vi "WaitForReceipt.vi"(8 "error in (no error)":errorcluster, 9 "timeout in ms (10000)":i32=10000, 11 "STOMP in":refnum<class "STOMP.lvclass">) -> (0 "error out":errorcluster, 2 "receipt":T1, 3 "STOMP out":refnum<class "STOMP.lvclass">)   [LabVIEW 2017, in "LabVIEW STOMP.lvlib" / "STOMP.lvclass"]
uses:
  STOMP.lvclass
  Typedefs/Type_ServerFrame.ctl
  Typedefs/Type_ServerFrameType.ctl
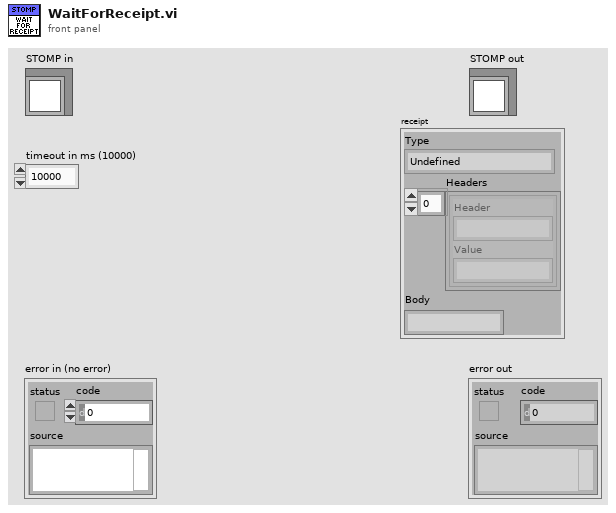
[diagram p1: front panel]
types:
  T1 = typedef "LabVIEW STOMP.lvlib/STOMP.lvclass/Type_ServerFrame.ctl" = cluster{"Type":T2, "Headers":cluster{"Header":string, "Value":string}[], "Body":string}
  T2 = typedef "LabVIEW STOMP.lvlib/STOMP.lvclass/Type_ServerFrameType.ctl" = enum16{"Undefined", "MESSAGE", "CONNECTED", "RECEIPT", "ERROR"}
  T3 = typedef "STOMP Connection Manager.lvclass/ObjectAttributes.ctl" = cluster{"address":string, "port":u16, "ConnectionRef":refnum<k5>, "messageQueue":refnum<queue>, "receiptQueue":refnum<queue>, "errorQueue":refnum<queue>, "sendQueue":refnum<queue>, "currentReceiptNumber":u64, "currentSubscriptionId":u64, "closeConnection":bool, "activeSubscriptions":T4[]}
  T4 = typedef "LabVIEW STOMP.lvlib/STOMP.lvclass/Type_ActiveSubscription.ctl" = cluster{"id":u64, "receipt":bool, "Destination":string, "ack":T5, "headers":T6[]}
  T5 = typedef "LabVIEW STOMP.lvlib/STOMP.lvclass/Type_AckHeader.ctl" = enum16{"auto", "client", "client-individual"}
  T6 = typedef "LabVIEW STOMP.lvlib/STOMP.lvclass/Type_FrameHeader.ctl" = cluster{"Header":string, "Value":string}
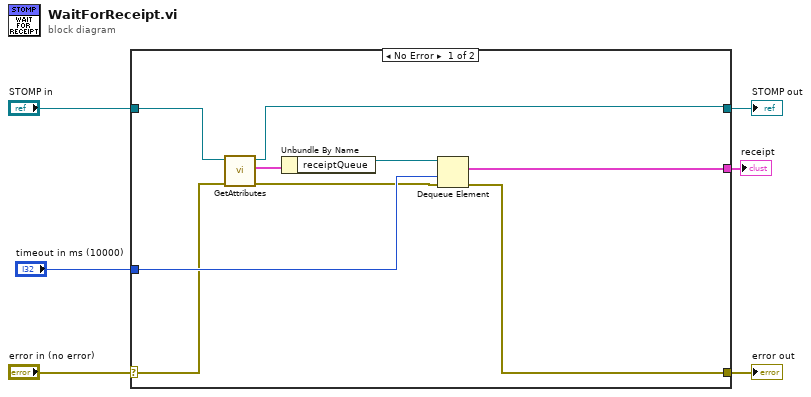
[diagram p0: block diagram]
diagram:
  n1 = case shown="No Error" "error in (no error)" {
    selector: "error in (no error)" -> [w8 w17]
    tunnel: [w12 w17] -> w5
    tunnel: [w9 w16] -> w3
    tunnel: "STOMP in" -> [w11 w16]
    tunnel: "timeout in ms (10000)" -> [w14 _]
    tunnel: [w13 _] -> w1
    frame No Error {
      n2 = call-dynamic "GetAttributes.vi"("error in (no error)"=w8, "STOMP in"=w11) -> ("error out"=w7:errorcluster, "attributes"=w10:T3, "STOMP out"=w9:refnum<class "STOMP.lvclass">)  [unwired: 7 in]
      n3 = Unbundle By Name(w10) -> ("receiptQueue"=w15:refnum<queue>)
      n4 = Dequeue Element(queue=w15, timeout in ms (-1)=w14, error in (no error)=w7) -> (element=w13:T1, error out=w12:errorcluster)  [unwired: 2 out]
    }
    frame Error {
    }
  }
  "error out" <- w5
  "STOMP out" <- w3
  "receipt" <- w1
